vi "Read Max Number of Cores.vi"(8 "error in (no error)":errorcluster, 11 "PC in":refnum<class "PC.lvclass">) -> (0 "error out":errorcluster, 2 "Max Number of Cores":dbl, 3 "PC out":refnum<class "PC.lvclass">)   [LabVIEW 2017, in "PC.lvclass"]
uses:
  PC.lvclass
  PC.lvclass/PC.ctl
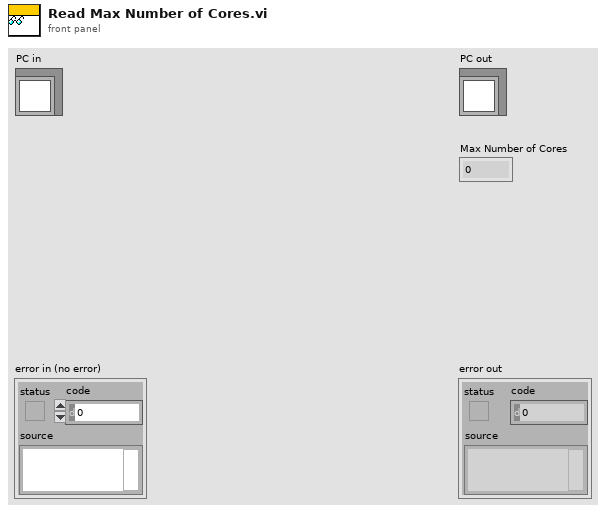
[diagram p1: front panel]
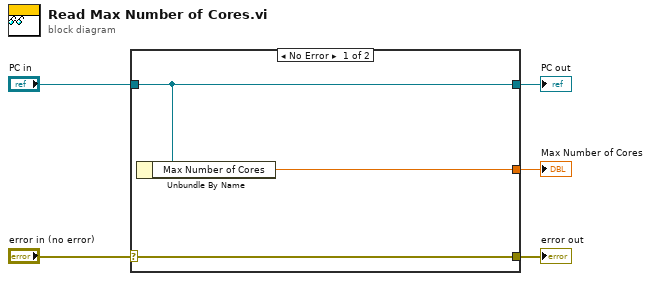
[diagram p0: block diagram]
diagram:
  n1 = case shown="No Error" "error in (no error)" {
    selector: "error in (no error)" -> [w8 w9]
    tunnel: [w8 w9] -> w4
    tunnel: [w7 w10] -> w2
    tunnel: "PC in" -> [w7 w10]
    tunnel: [w6 _] -> w1
    frame No Error {
      n2 = Unbundle By Name(w7) -> ("Max Number of Cores"=w6:dbl)
    }
    frame Error {
    }
  }
  "error out" <- w4
  "PC out" <- w2
  "Max Number of Cores" <- w1
